vi "ConvertCircleToBoundingBox.vi"(8 "error in (no error)":errorcluster, 9 "InflateBoxbyPixelNo":dbl=3.0, 10 "Radius":dbl, 11 "Position":cluster{"X":sgl, "Y":sgl}) -> (0 "error out":errorcluster, 3 "Bounding Box":cluster{"x":sgl, "y":sgl}[](array[cluster]))   [LabVIEW 2015]
doc: "Use this template to build a VI to use as a subVI."
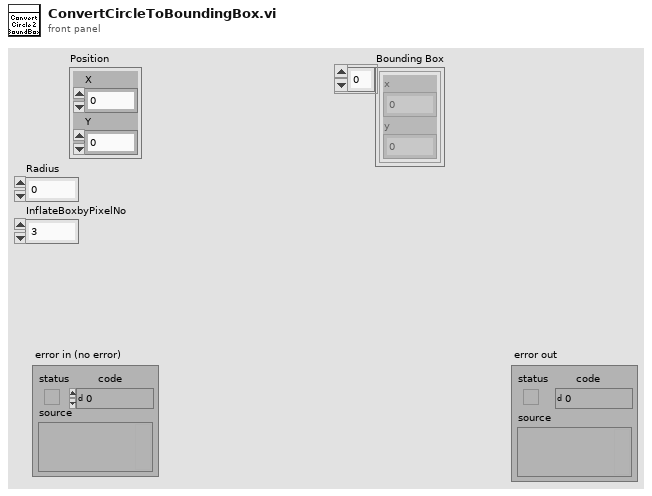
[diagram p1: front panel]
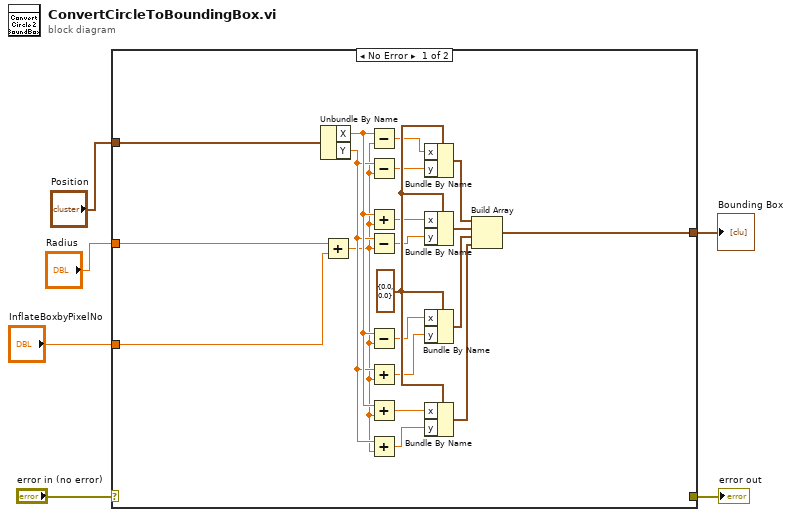
[diagram p0: block diagram]
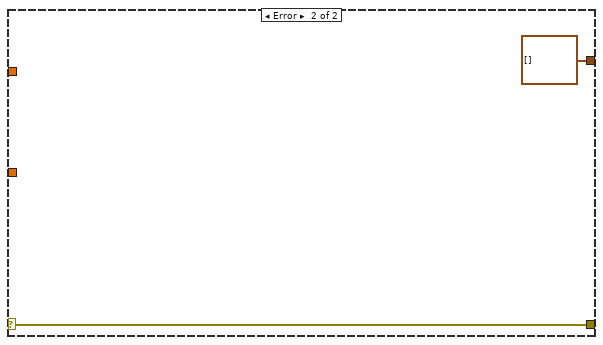
[diagram p2: hidden frame]
diagram:
  n1 = case shown="No Error" "error in (no error)" {
    selector: "error in (no error)" -> [_ w28]
    tunnel: [_ w28] -> w5
    tunnel: "Position" -> [w10 _]
    tunnel: "Radius" -> [w9 _]
    tunnel: "InflateBoxbyPixelNo" -> [w8 _]
    tunnel: [w7 cluster{"x":sgl, "y":sgl}[] []] -> w1
    frame No Error {
      w24 = cluster{"x":sgl, "y":sgl} {"x"=0.0, "y"=0.0} ("Position 2")
      n2 = Unbundle By Name(w10) -> ("X"=w15:sgl, "Y"=w14:sgl)
      n3 = Add(x=w9, y=w8) -> (x+y=w11:dbl)
      n4 = Subtract(x=w15, y=w11) -> (x-y=w21:dbl)
      n5 = Subtract(x=w14, y=w11) -> (x-y=w20:dbl)
      n6 = Add(x=w15, y=w11) -> (x+y=w19:dbl)
      n7 = Subtract(x=w14, y=w11) -> (x-y=w18:dbl)
      n8 = Subtract(x=w15, y=w11) -> (x-y=w17:dbl)
      n9 = Add(x=w14, y=w11) -> (x+y=w16:dbl)
      n10 = Add(x=w15, y=w11) -> (x+y=w13:dbl)
      n11 = Add(x=w14, y=w11) -> (x+y=w12:dbl)
      n12 = Bundle By Name(cluster=w24, "x"=w21, "y"=w20) -> (w26:cluster{"x":sgl, "y":sgl})
      n13 = Bundle By Name(cluster=w24, "x"=w19, "y"=w18) -> (w25:cluster{"x":sgl, "y":sgl})
      n14 = Bundle By Name(cluster=w24, "x"=w17, "y"=w16) -> (w23:cluster{"x":sgl, "y":sgl})
      n15 = Bundle By Name(cluster=w24, "x"=w13, "y"=w12) -> (w22:cluster{"x":sgl, "y":sgl})
      n16 = Build Array(w26, w25, w23, w22) -> (w7:cluster{"x":sgl, "y":sgl}[])
    }
    frame Error {
    }
  }
  "error out" <- w5
  "Bounding Box" <- w1
